vi "Pack for gRPC.vi"(8 "error in":errorcluster, 9 "configuration / results":enum16{"Configuration", "Results"}(ring), 10 "data value":variant, 11 "measurement customizations in":refnum<class "Measurement Plugin.lvclass">) -> (0 "error out":errorcluster, 2 "any":T1, 3 "measurement customizations out":refnum<class "Measurement Plugin.lvclass">)   [LabVIEW 2024, in "OneShot-PureTone.lvlib" / "Measurement Plugin.lvclass"]
uses:
  Measurement Plugin.lvclass
  <vilib>/gRPC/LabVIEW gRPC Library/Shared/Any.ctl
  C:/Program Files/National Instruments/LabVIEW 2024/vi.lib/Plug-In SDKs/Measurements/Measurement Plugin Service/Measurement Plugin Service.lvclass
  Measurement Configuration.ctl
  Measurement Results.ctl
  2eca732d-dbaa-43bf-a7dd-ede2da65bc1b.vi
  a6012965-5700-4384-8228-972e71b6560c.vi
  <vilib>/gRPC/LabVIEW gRPC Library/Server API/Translate Protobuf Error.vi
  <vilib>/AdvancedString/1D String Array to Delimited String.vi
  <vilib>/gRPC/LabVIEW gRPC Library/Server API/Server/Get Server DLL Path.vi
  OneShot-PureTone.lvlib
  <vilib>/Plug-In SDKs/Measurements/Measurement Plugin Service/Measurement Plugin Service.lvclass
  <vilib>/gRPC/LabVIEW gRPC Library/grpc-lvsupport-release.lvlib
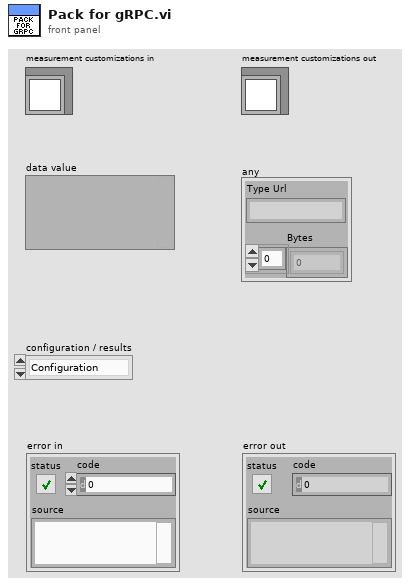
[diagram p1: front panel]
types:
  T1 = typedef "grpc-lvsupport-release.lvlib/Any.ctl" = cluster{"Type Url":string, "Bytes":u8[]}
  T2 = typedef "grpc-lvsupport-release.lvlib/grpcId.ctl" = u64
  T3 = typedef "OneShot-PureTone.lvlib/Measurement Configuration.ctl" = cluster{"THD maximum harmonic":i32, "measurement duration (s)":dbl, "measurement cycles":dbl, "band start (Hz)":dbl, "band stop (Hz)":dbl, "settle time (s)":dbl, "settle cycles":dbl, "AI range":dbl, "output channel":string, "input channel":string, "frequency (Hz)":dbl, "amplitude":dbl, "sample rate (Hz)":dbl}
  T4 = typedef "OneShot-PureTone.lvlib/Measurement Results.ctl" = cluster{"band start (Hz) out":dbl, "band stop (Hz) out":dbl, "detected frequency (Hz)":dbl, "detected amplitude":dbl, "acquired response":dbl[], "measurement subset":dbl[], "acquired response t0":dbl, "acquired response dt":dbl, "measurement subset t0":dbl, "measurement subset dt":dbl, "THD maximum harmonic out":i32}
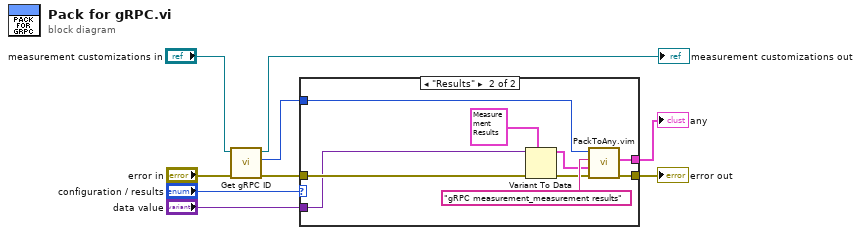
[diagram p0: block diagram]
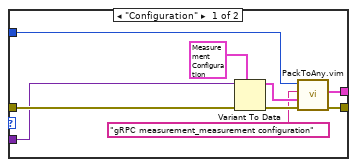
[diagram p2: hidden frame]
diagram:
  n1 = call <vilib>:"Get gRPC ID.vi"("error in"="error in", "measurement plugin service in"="measurement customizations in") -> ("error out"=w4:errorcluster, "gRPC ID"=w1:T2, "measurement plugin service out"=→"measurement customizations out":refnum<class "Measurement Plugin.lvclass">)  [unwired: 7 in]
  n2 = case shown="\"Results\"" "configuration / results" {
    tunnel: w4 -> [w18 w27]
    tunnel: "data value" -> [w17 w26]
    tunnel: w1 -> [w14 w22]
    tunnel: [w16 w24] -> w8
    tunnel: [w15 w23] -> w7
    frame "Configuration" {
      n3 = Variant To Data(error in=w18, type=T3 {"THD maximum harmonic"=1, "measurement duration (s)"=1.2, "measurement cycles"=32.0, "band start (Hz)"=32.0, "band stop (Hz)"=64.0, "settle time (s)"=-32.0, "settle cycles"=-64.0, "AI range"=-64.0, "output channel"="Lorem ipsum dolor sit", "input channel"="Dev1/ai0", "frequency (Hz)"=1.0, "amplitude"=1.0, "sample rate (Hz)"=51200.0} ("measurement configuration"), Variant=w17) -> (data=w13:T3, error out=w12:errorcluster)
      n4 = call "PackToAny.vim"("error in"=w12, "Data To Pack"=w13, "Message Type"="gRPC measurement_measurement configuration", "gRPCid in"=w14) -> ("error out"=w16:errorcluster, "Any"=w15:T1)  [unwired: 5 in, 1 out]
    }
    frame "Results" {
      n5 = Variant To Data(error in=w27, type=T4 {"band start (Hz) out"=0.0, "band stop (Hz) out"=0.0, "detected frequency (Hz)"=0.0, "detected amplitude"=0.0, "acquired response"=[], "measurement subset"=[], "acquired response t0"=0.0, "acquired response dt"=0.0, "measurement subset t0"=0.0, "measurement subset dt"=0.0, "THD maximum harmonic out"=9} ("Measurement Results"), Variant=w26) -> (data=w20:T4, error out=w19:errorcluster)
      n6 = call "PackToAny.vim"("error in"=w19, "Data To Pack"=w20, "Message Type"="gRPC measurement_measurement results", "gRPCid in"=w22) -> ("error out"=w24:errorcluster, "Any"=w23:T1)  [unwired: 5 in, 1 out]
    }
  }
  "error out" <- w8
  "any" <- w7
